vi "Read Next Message.vi"(0 "message queue in":T3, 1 "ignore error on termination message (F)":bool, 7 "termination list ([Exit])":string[](array[string])=["Exit"], 9 "timeout (1 ms)":i32=1, 11 "error in":errorcluster) -> (3 "exit process?":bool, 4 "message queue out":T3, 6 "message name":string, 8 "message value":string, 10 "timed out?":bool, 13 "acknowledge":bool, 14 "message":T1, 15 "error out":errorcluster)   [LabVIEW 2009, in "AMC.lvlib"]
doc: "Returns the next message from the message queue passed in. If the returned message matches any of the message names listed in \"termination list\" the \"exit process?\" indicator will return True."
uses:
  AMC.lvlib
  Message Queue.ctl
  Message.ctl
  <vilib>/NI/Tools/Keyed Array/KeyedArray.ctl
  Globals.vi
  <vilib>/NI/Tools/Keyed Array/Tools_KeyedArray.lvlib
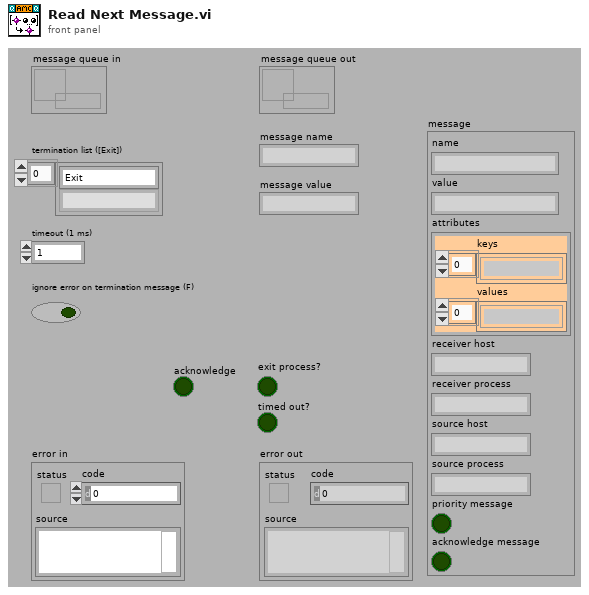
[diagram p1: front panel]
types:
  T1 = typedef "AMC.lvlib/Message.ctl" = cluster{"name":string, "value":string, "attributes":T2, "receiver host":string, "receiver process":string, "source host":string, "source process":string, "priority message":bool, "acknowledge message":bool}
  T2 = typedef "Tools_KeyedArray.lvlib/KeyedArray.ctl" = cluster{"keys":string[], "values":string[]}
  T3 = typedef "AMC.lvlib/Message Queue.ctl" = refnum<queue>
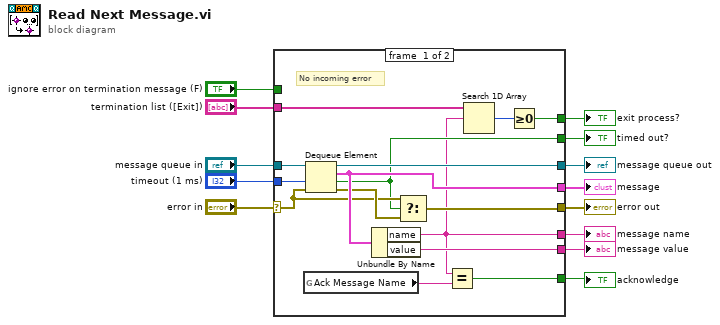
[diagram p0: block diagram]
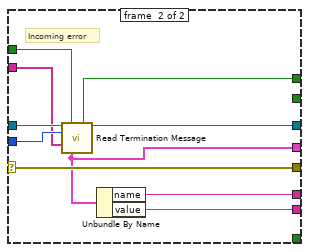
[diagram p2: hidden frame]
diagram:
  n1 = case shown="No Error" "error in" {
    selector: "error in" -> [w19 w32]
    tunnel: "message queue in" -> [w28 w38]
    tunnel: [w27 w34] -> w11
    tunnel: [w15 w30] -> w13
    tunnel: "timeout (1 ms)" -> [w26 w37]
    tunnel: [w20 w32] -> w12
    tunnel: [w17 w29] -> w10
    tunnel: [w25 w31] -> w9
    tunnel: "termination list ([Exit])" -> [w24 w35]
    tunnel: [w22 w33] -> w8
    tunnel: "ignore error on termination message (F)" -> [_ w36]
    tunnel: [w18 _] -> w2
    tunnel: [w14 _] -> w1
    frame #0 {
      # "No incoming error"
      n2 = global read "Globals.vi" "Ack Message Name"() -> (w16:string)
      n3 = Dequeue Element(queue=w28, timeout in ms (-1)=w26, error in (no error)=w19) -> (queue out=w27:T3, element=w25:T1, timed out?=w18:bool, error out=w21:errorcluster)
      n4 = Unbundle By Name(w25) -> ("name"=w15:string, "value"=w17:string)
      n5 = Select(t=w19, s=w18, f=w21) -> (s? t:f=w20:errorcluster)
      n6 = Equal?(x=w15, y=w16) -> (x = y?=w14:bool)
      n7 = Search 1D Array(1D array=w24, element=w15) -> (index of element=w23:i32)  [unwired: 1 out]
      n8 = Greater Or Equal To 0?(x=w23) -> (x >= 0?=w22:bool)
    }
    frame #1 {
      # "Incoming error"
      n9 = call "Read Termination Message.vi"("message queue in"=w38, "ignore error on termination message (F)"=w36, "timeout (1 ms)"=w37, "termination list ([Exit])"=w35) -> ("termination message"=w33:bool, "message queue out"=w34:T3, "message"=w31:T1)  [unwired: 9 in]
      n10 = Unbundle By Name(w31) -> ("name"=w30:string, "value"=w29:string)
    }
  }
  "message queue out" <- w11
  "message name" <- w13
  "error out" <- w12
  "message value" <- w10
  "message" <- w9
  "exit process?" <- w8
  "timed out?" <- w2
  "acknowledge" <- w1
